vi "ReturnMovePattern.vi"(8 "error in (no error)":errorcluster, 11 "object in":refnum<class "Bishop.lvclass">) -> (0 "error out":errorcluster, 3 "object out":refnum<class "Bishop.lvclass">)   [LabVIEW 2020, in "Bishop.lvclass"]
uses:
  Bishop.lvclass
  C:/_repos/_personal/Chess/Chess_LV/src/source/Pieces/Piece.lvclass
  Piece.lvclass
panel:
  out "Array":map{string, i32}[](array[numeric])
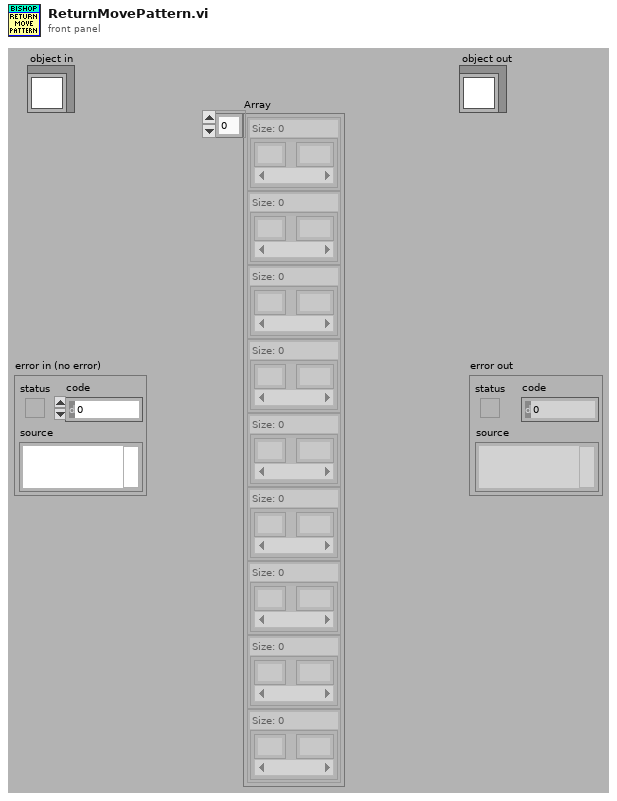
[diagram p1: front panel]
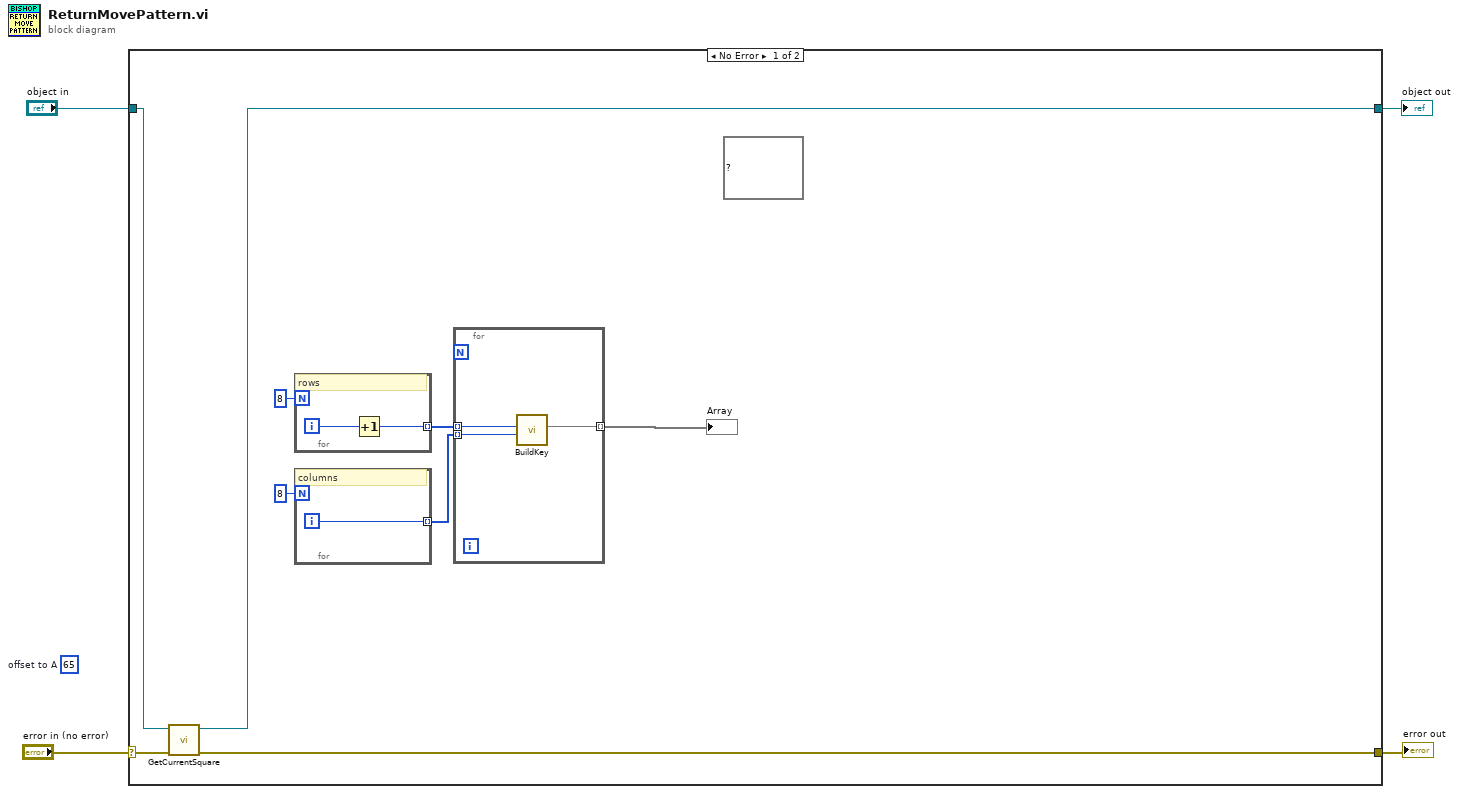
[diagram p0: block diagram]
diagram:
  (unwired) 65  # offset to A
  n1 = case shown="No Error" "error in (no error)" {
    selector: "error in (no error)" -> [w13 w21]
    tunnel: [w12 w21] -> w3
    tunnel: [w9 w20] -> w1
    tunnel: "object in" -> [w11 w20]
    frame No Error {
      (unwired) map{string, i32} {"H"=1} ("currentSquare")
      n2 = call "GetCurrentSquare.vi"("error in (no error)"=w13, "object in"=w11) -> ("error out"=w12:errorcluster, "object out"=w9:refnum<class "Bishop.lvclass">)  [unwired: 4 in, 4 out]
      n3 = for {
        N: 8 -> [_]
        tunnel: [w17] -> w7 mode=indexing
        i -> [w18]
        # "rows"
        n4 = Increment(x=w18) -> (x+1=w17:i32)
      }
      n5 = for {
        N: 8 -> [_]
        tunnel: [w19] -> w6 mode=indexing
        i -> [w19]
        # "columns"
      }
      n6 = for {
        tunnel: w7 -> [w16] mode=indexing
        tunnel: w6 -> [w15] mode=indexing
        tunnel: [w14] -> w5 mode=indexing
        n7 = call "BuildKey.vi"("Column (65=A)"=w15, "Row (>=1)"=w16) -> ("Built Key"=w14:map{string, i32})  [unwired: 7 in, 2 out]
      }
      "Array" <- w5
    }
    frame Error {
    }
  }
  "error out" <- w3
  "object out" <- w1
